vi "Open New Email Msg.vi"(8 "error in (no error)":errorcluster, 9 "Body":string="Describe your problem.", 10 "Subject":string="System Complications", 11 "Recipient":string="pysz@student.agh.edu.pl") -> (0 "error out":errorcluster)   [LabVIEW 2021]
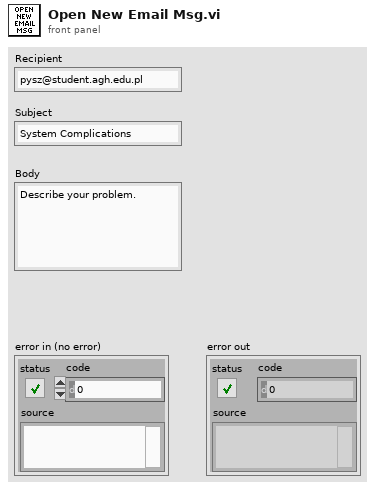
[diagram p1: front panel]
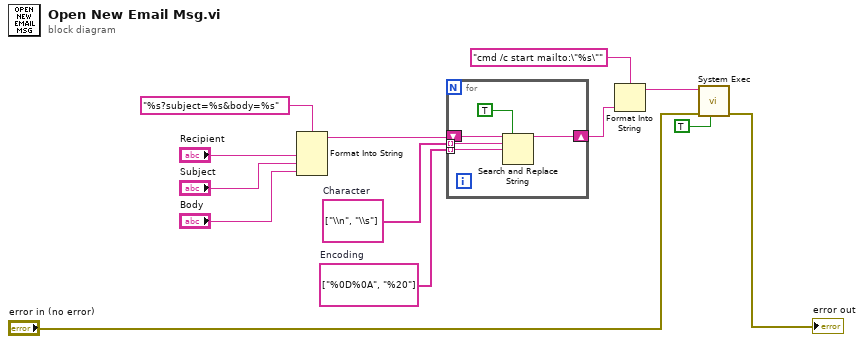
[diagram p0: block diagram]
diagram:
  w11 = string[] ["%0D%0A", "%20"]  # Encoding
  w12 = string[] ["\\n", "\\s"]  # Character
  n1 = Format Into String(format string="%s?subject=%s&body=%s", "Recipient", "Subject", "Body") -> (resulting string=w6:string)  [unwired: 2 in, 1 out]
  n2 = for {
    shift-right: [w17] -> w5
    shift-left: w6 -> [w16]
    tunnel: w11 -> [w15] mode=indexing
    tunnel: w12 -> [w14] mode=indexing
    n3 = Search and Replace String(replace all?=TRUE ("replace all? (F)"), input string=w16, search string=w14, replace string=w15) -> (result string=w17:string)  [unwired: 4 in, 3 out]
  }
  n4 = Format Into String(format string="cmd /c start mailto:\"%s\"", w5) -> (resulting string=w4:string)  [unwired: 2 in, 1 out]
  n5 = call <vilib>:"System Exec.vi"("run minimized? (F)"=TRUE, "error in (no error)"="error in (no error)", "command line"=w4) -> ("error out"=→"error out":errorcluster)  [unwired: 5 in, 3 out]
